vi "Init Last Readings Buffer.vi"(8 "error in":errorcluster, 11 "BufferLastReadingsDBL in":refnum<class "BufferLastReadsDBL.lvclass">) -> (0 "error out":errorcluster, 3 "BufferLastReadingsDBL out":refnum<class "BufferLastReadsDBL.lvclass">)   [LabVIEW 2024]
uses:
  BufferLastReadsDBL.lvclass/BufferLastReadsDBL.ctl
  BufferLastReadsDBL.lvclass
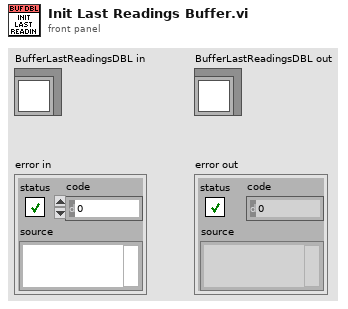
[diagram p1: front panel]
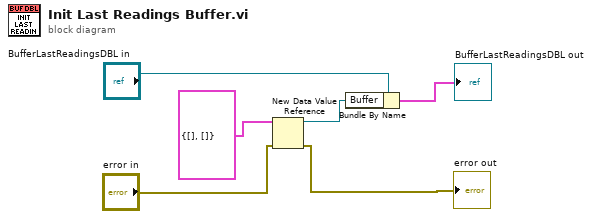
[diagram p0: block diagram]
diagram:
  n1 = New Data Value Reference(data value=cluster{"Idents":string[], "Readings":dbl[]} {"Idents"=[], "Readings"=[]}, error in="error in") -> (data value reference=w1:refnum<data-value>, error out=→"error out":errorcluster)
  n2 = Bundle By Name(cluster="BufferLastReadingsDBL in", "Buffer"=w1) -> (→"BufferLastReadingsDBL out":cluster{})
